vi "Polar - Mark Label.vi"(10 "Position":cluster{i16, i16}[](array[cluster]), 11 "new picture in":picture) -> (3 "new picture":picture)   [LabVIEW 2020]
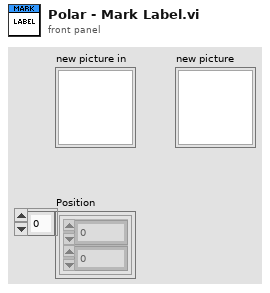
[diagram p1: front panel]
types:
  T1 = cluster{"Font Name:":string, "Size":i16, "Strikeout?":bool, "Italic?":bool, "Underline?":bool, "Outline?":bool, "Shadow?":bool, "Bold?":bool}
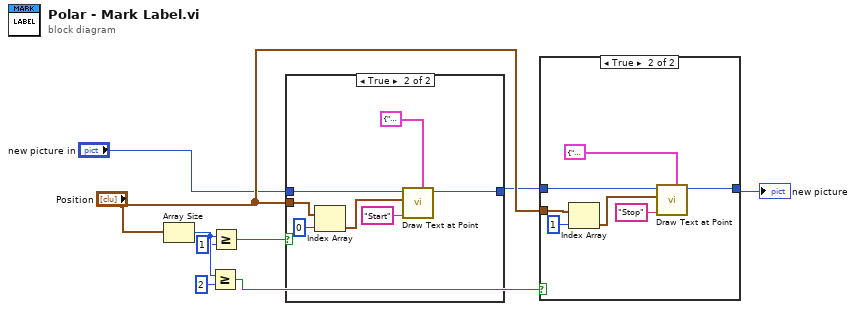
[diagram p0: block diagram]
diagram:
  n1 = Array Size(array="Position") -> (size(s)=w7:i32)
  n2 = Greater Or Equal?(x=w7, y=2) -> (x >= y?=w8:bool)
  n3 = Greater Or Equal?(x=w7, y=1) -> (x >= y?=w5:bool)
  n4 = case shown="True" w5 {
    tunnel: "new picture in" -> [w10 w17]
    tunnel: [w10 w16] -> w2
    tunnel: "Position" -> [_ w13]
    frame False {
    }
    frame True {
      n5 = Index Array(array=w13, index=0) -> (element=w12:cluster{i16, i16})
      n6 = call <vilib>:"Draw Text at Point.vi"("[user-specified font]"=T1 {"Font Name:"="", "Size"=15, "Strikeout?"=FALSE, "Italic?"=FALSE, "Underline?"=FALSE, "Outline?"=FALSE, "Shadow?"=FALSE, "Bold?"=FALSE}, "text"="Start", "origin"=w12, "picture"=w17) -> ("new picture"=w16:picture)  [unwired: 6 in, 1 out]
    }
  }
  n7 = case shown="True" w8 {
    tunnel: w2 -> [w18 w25]
    tunnel: [w18 w24] -> w3
    tunnel: "Position" -> [_ w21]
    frame False {
    }
    frame True {
      n8 = Index Array(array=w21, index=1) -> (element=w20:cluster{i16, i16})
      n9 = call <vilib>:"Draw Text at Point.vi"("[user-specified font]"=T1 {"Font Name:"="", "Size"=15, "Strikeout?"=FALSE, "Italic?"=FALSE, "Underline?"=FALSE, "Outline?"=FALSE, "Shadow?"=FALSE, "Bold?"=FALSE}, "text"="Stop", "origin"=w20, "picture"=w25) -> ("new picture"=w24:picture)  [unwired: 6 in, 1 out]
    }
  }
  "new picture" <- w3
